vi "FP add waypoints.vi"(2 "error in":errorcluster, 3 "MDF Control":T1(array[cluster]), 4 "Image In":T2) -> (0 "error out":errorcluster, 1 "Image Out":T2)   [LabVIEW 2014]
doc: "This vi will overlay the waypoints created in the Mission Definition File onto the pool image."
uses:
  <vilib>/vision/Image Controls.llb/IMAQ Image.ctl
panel:
  out "size(s)":i32
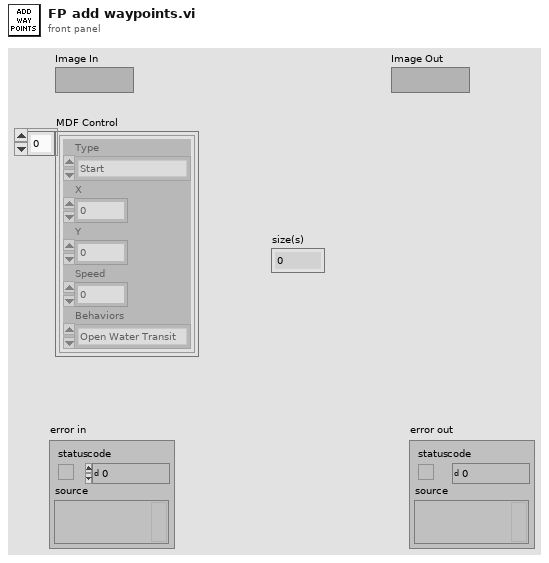
[diagram p1: front panel]
types:
  T1 = cluster{"Type":enum16{"Start", "Waypoint", "End"}, "X":i32, "Y":i32, "Speed":i32, "Behaviors":enum16{"Open Water Transit", "P-Wall Follow", "S-Wall Follow", "Dock"}}[]
  T2 = typedef "IMAQ Image.ctl" = refnum<image>
  T3 = cluster{"Desired Font (Application)":enum16{"User-specified Font", "Application Font", "System Font", "Dialog Font"}, "[User-specified Font]":cluster{"Font Name":string, "Size":i16, "Strikeout?":bool, "Italic?":bool, "Underline?":bool, "Outline?":bool, "Shadow?":bool, "Bold?":bool, "Rotation Angle":dbl}, "Horizontal Alignment":i16, "Vertical Alignment":i16}
  T4 = cluster{"Type":enum16{"Start", "Waypoint", "End"}, "X":i32, "Y":i32, "Speed":i32, "Behaviors":enum16{"Open Water Transit", "P-Wall Follow", "S-Wall Follow", "Dock"}}
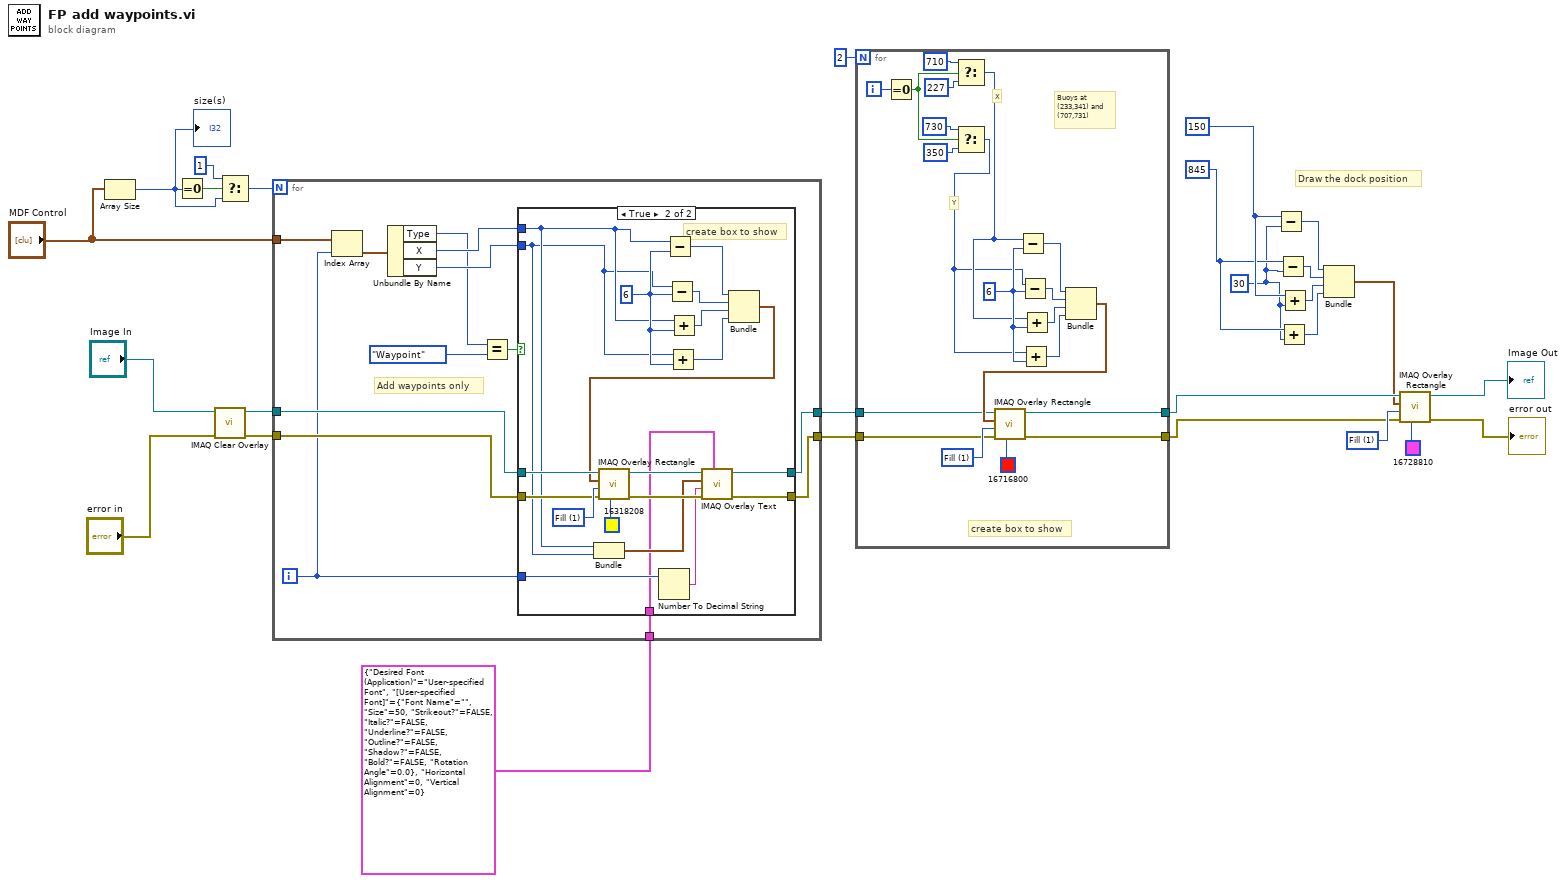
[diagram p0: block diagram]
diagram:
  w1 = 30 ("t")
  w2 = 845 ("t")
  w3 = 150 ("t")
  w14 = u32 1 items=["Frame", "Fill", "Highlight"] ("Drawing Mode (Frame)")
  # "Draw the dock position"
  n1 = Array Size(array="MDF Control") -> (size(s)=w20:i32)
  "size(s)" <- w20
  n2 = Equal To 0?(x=w20) -> (x = 0?=w23:bool)
  n3 = call "IMAQ Clear Overlay"("error in (no error)"="error in", "Image"="Image In") -> ("error out"=w26:errorcluster, "Image Out"=w24:T2)  [unwired: 8 in]
  n4 = Select(t=1, s=w23, f=w20) -> (s? t:f=w21:i32)
  n5 = for {
    N: w21 -> [_]
    tunnel: [w40] -> w18
    tunnel: [w39] -> w17
    tunnel: w26 -> [w38]
    tunnel: w24 -> [w37]
    tunnel: "MDF Control" -> [w36]
    tunnel: T3 {"Desired Font (Application)"=enum."User-specified Font", "[User-specified Font]"={"Font Name"="", "Size"=50, "Strikeout?"=FALSE, "Italic?"=FALSE, "Underline?"=FALSE, "Outline?"=FALSE, "Shadow?"=FALSE, "Bold?"=FALSE, "Rotation Angle"=0.0}, "Horizontal Alignment"=0, "Vertical Alignment"=0} ("Font, Size & Style") -> [w28]
    i -> [w29]
    # "Add waypoints only"
    n6 = Index Array(array=w36, index=w29) -> (element=w35:T4)
    n7 = Unbundle By Name(w35) -> ("Type"=w31:enum16{"Start", "Waypoint", "End"}, "X"=w34:i32, "Y"=w33:i32)
    n8 = Equal?(x=w31, y=enum16{"Start", "Waypoint", "End"}."Waypoint" ("Type")) -> (x = y?=w32:bool)
    n9 = case shown="True" w32 {
      tunnel: [w42 w51] -> w40
      tunnel: [w41 w49] -> w39
      tunnel: w38 -> [w41 w60]
      tunnel: w37 -> [w42 w59]
      tunnel: w34 -> [_ w46]
      tunnel: w33 -> [_ w45]
      tunnel: w29 -> [_ w48]
      tunnel: w28 -> [_ w43]
      frame False {
      }
      frame True {
        w58 = 6
        w61 = u32 1 items=["Frame", "Fill", "Highlight"] ("Drawing Mode (Frame)")
        # "create box to show"
        n10 = Bundle("X"=w46, "Y"=w45) -> (w44:cluster{"X":i32, "Y":i32})  [unwired: 1 in]
        n11 = Number To Decimal String(number=w48) -> (decimal integer string=w47:string)  [unwired: 1 in]
        n12 = Subtract(x=w46, y=w58) -> (x-y=w57:i32)
        n13 = Subtract(x=w45, y=w58) -> (x-y=w56:i32)
        n14 = Add(x=w45, y=w58) -> (x+y=w54:i32)
        n15 = Add(x=w46, y=w58) -> (x+y=w55:i32)
        n16 = Bundle(w57, w56, w55, w54) -> (w53:cluster{i32, i32, i32, i32})  [unwired: 1 in]
        n17 = call "IMAQ Overlay Rectangle"("Color"=u32 16318208, "error in (no error)"=w60, "Drawing Mode (Frame)"=w61, "Rectangle"=w53, "Image"=w59) -> ("error out"=w50:errorcluster, "Image Out"=w52:T2)  [unwired: 5 in]
        n18 = call "IMAQ Overlay Text"("Font, Size & Style"=w43, "error in (no error)"=w50, "String"=w47, "Origin"=w44, "Image"=w52) -> ("error out"=w49:errorcluster, "Image Out"=w51:T2)  [unwired: 5 in]
      }
    }
  }
  n19 = for {
    N: 2 -> [_]
    tunnel: w18 -> [w74]
    tunnel: [w63] -> w10
    tunnel: w17 -> [w73]
    tunnel: [w64] -> w12
    i -> [w65]
    w80 = 6
    w81 = u32 1 items=["Frame", "Fill", "Highlight"] ("Drawing Mode (Frame)")
    # "Buoys at \n(233,341) and \n(707,731)"
    # "Y"
    # "X"
    # "create box to show"
    n20 = Equal To 0?(x=w65) -> (x = 0?=w72:bool)
    n21 = Select(t=710, s=w72, f=227 ("t")) -> (s? t:f=w67:i32)
    n22 = Select(t=730, s=w72, f=350 ("t")) -> (s? t:f=w66:i32)
    n23 = Subtract(x=w67, y=w80) -> (x-y=w79:i32)
    n24 = Subtract(x=w66, y=w80) -> (x-y=w78:i32)
    n25 = Add(x=w66, y=w80) -> (x+y=w76:i32)
    n26 = Add(x=w67, y=w80) -> (x+y=w77:i32)
    n27 = Bundle(w79, w78, w77, w76) -> (w75:cluster{i32, i32, i32, i32})  [unwired: 1 in]
    n28 = call "IMAQ Overlay Rectangle"("Color"=u32 16716800, "error in (no error)"=w73, "Drawing Mode (Frame)"=w81, "Rectangle"=w75, "Image"=w74) -> ("error out"=w64:errorcluster, "Image Out"=w63:T2)  [unwired: 5 in]
  }
  n29 = Subtract(x=w3, y=w1) -> (x-y=w5:i32)
  n30 = Subtract(x=w2, y=w1) -> (x-y=w6:i32)
  n31 = Add(x=w2, y=w1) -> (x+y=w8:i32)
  n32 = Add(x=w3, y=w1) -> (x+y=w7:i32)
  n33 = Bundle(w5, w6, w7, w8) -> (w4:cluster{i32, i32, i32, i32})  [unwired: 1 in]
  n34 = call "IMAQ Overlay Rectangle"("Color"=u32 16728810, "error in (no error)"=w12, "Drawing Mode (Frame)"=w14, "Rectangle"=w4, "Image"=w10) -> ("error out"=→"error out":errorcluster, "Image Out"=→"Image Out":T2)  [unwired: 5 in]
